vi "ProcessModbusUpdates.vi"(11 "MockInclinSettings":T1={"ModbusRxDataFIFO"="ModbusInclinRxDataFIFO", "ModbusTxDataFIFO"="ModbusInclinTxDataFIFO", "BufferUpdateFIFO"="MockInclinCommand", "InclinAngleMemory"="MockInlcinAngle"}) -> ()   [LabVIEW 2016]
uses:
  FPGAMockHPILC/DataTypes/MockHPModbusUpdateStates.ctl
  FPGAMockHPILC/FPGAMockHPILC.lvlib
  FPGAMockHPILC/DataTypes/MockHPModbusUpdateLoopData.ctl
  <vilib>/rvi/DataTransferAndStorage/Container/XNode/niFpgaContainer.xnode
  <vilib>/rvi/FIFO/Fifo_Resource/niFpgaFifoEmulationRefIn.vi
  <vilib>/rvi/FIFO/Fifo_Resource/nirvififoEmulationWrite.vi
  <vilib>/rvi/Memory/Memory_Emulation/nirvimemoryFastEmulation.vi
  <vilib>/rvi/Memory/Memory_Emulation/nirvimemoryEmulation.vi
  <vilib>/rvi/FIFO/Fifo_Resource/nirvififoEmulationRead.vi
  <vilib>/eio/EIOMethodNode/EIOMethodNode.xnode
  <vilib>/rvi/eio/common/nirviEmuTemplateMethod_errors.vi
  DataTypes/MockInclinSettings.ctl
  FPGAMockInclin.lvlib
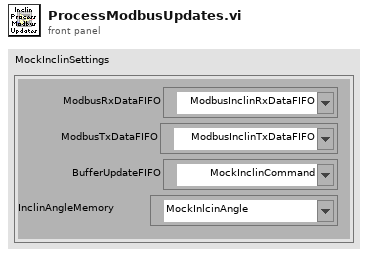
[diagram p1: front panel]
types:
  T1 = typedef "FPGAMockInclin.lvlib/MockInclinSettings.ctl" = cluster{"ModbusRxDataFIFO":refnum<k21>, "ModbusTxDataFIFO":refnum<k21>, "BufferUpdateFIFO":refnum<k21>, "InclinAngleMemory":refnum<k21>}
  T2 = typedef "FPGAMockHPILC.lvlib/MockHPModbusUpdateLoopData.ctl" = cluster{"ModbusUpdateLoopStates":T3, "Address":u8, "Function":u8, "ResponseLength":u8, "ResponseIndex":u8, "Index":u8, "Data":u16, "DelayTicks":u32}
  T3 = typedef "FPGAMockHPILC.lvlib/MockHPModbusUpdateStates.ctl" = enum16{"ReadModbusPort", "ProcessModbusData", "DelayMicroseconds", "WriteAddress", "WriteFunction", "WriteData", "WriteCRCLSB", "WriteCRCMSB", "WriteEndOfFrame", "CalculateCRC"}
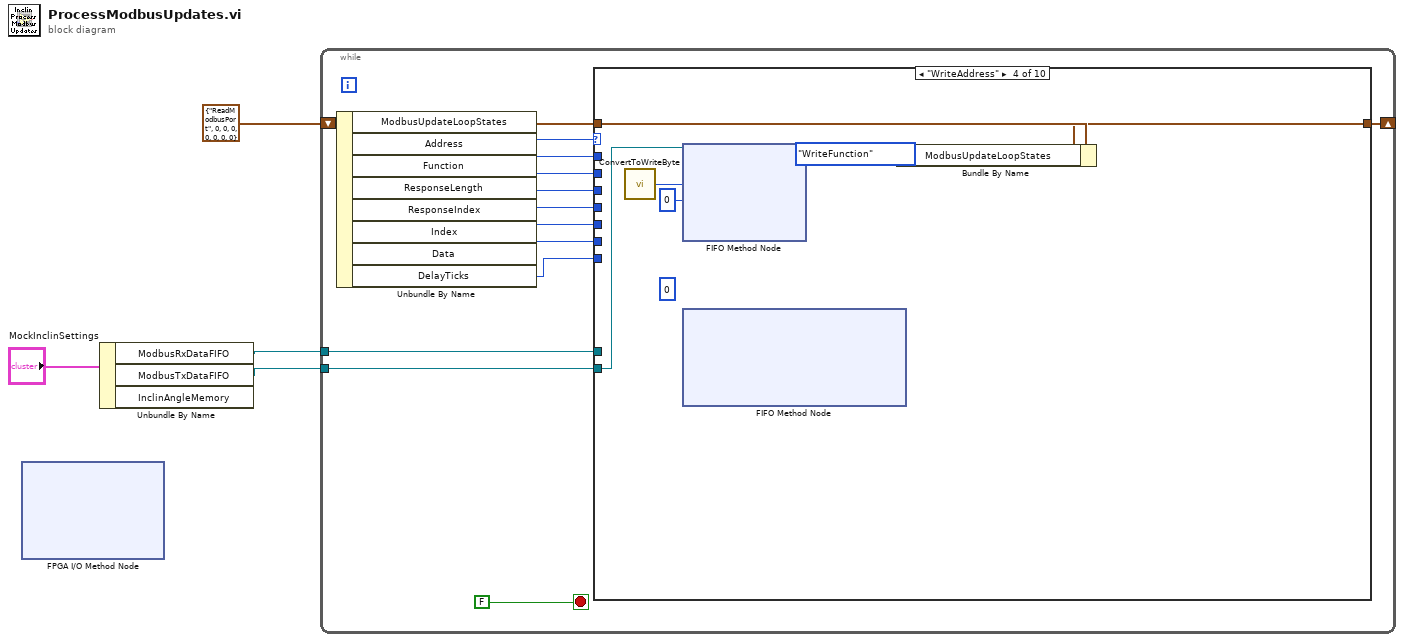
[diagram p0: block diagram]
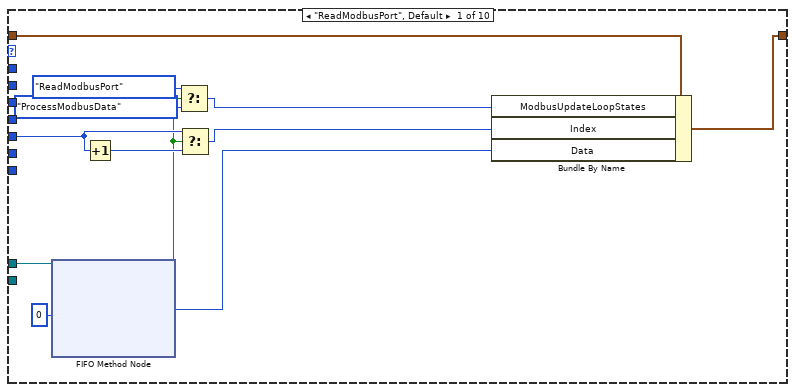
[diagram p2: hidden frame]
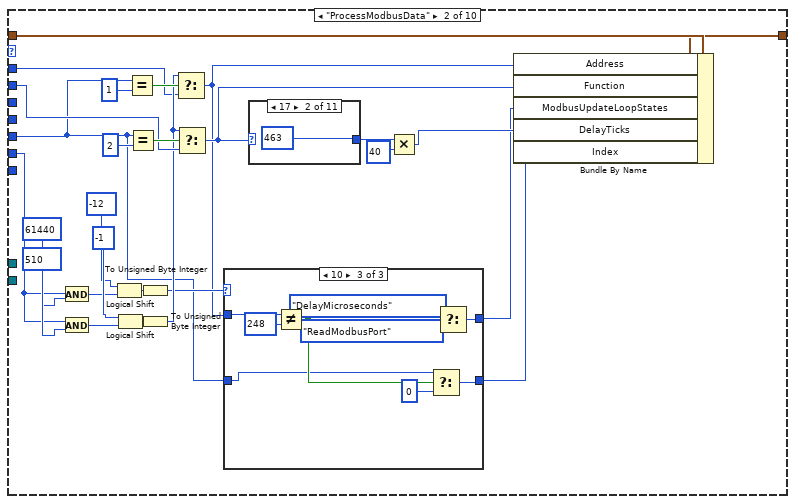
[diagram p3: hidden frame]
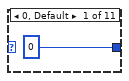
[diagram p4: hidden frame]
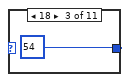
[diagram p5: hidden frame]
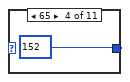
[diagram p6: hidden frame]
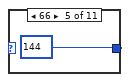
[diagram p7: hidden frame]
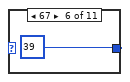
[diagram p8: hidden frame]
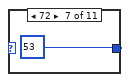
[diagram p9: hidden frame]
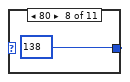
[diagram p10: hidden frame]
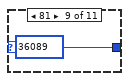
[diagram p11: hidden frame]
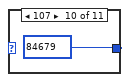
[diagram p12: hidden frame]
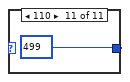
[diagram p13: hidden frame]
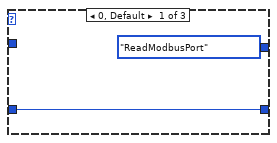
[diagram p14: hidden frame]
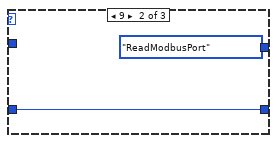
[diagram p15: hidden frame]
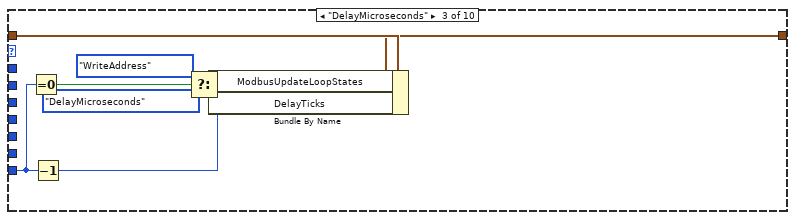
[diagram p16: hidden frame]
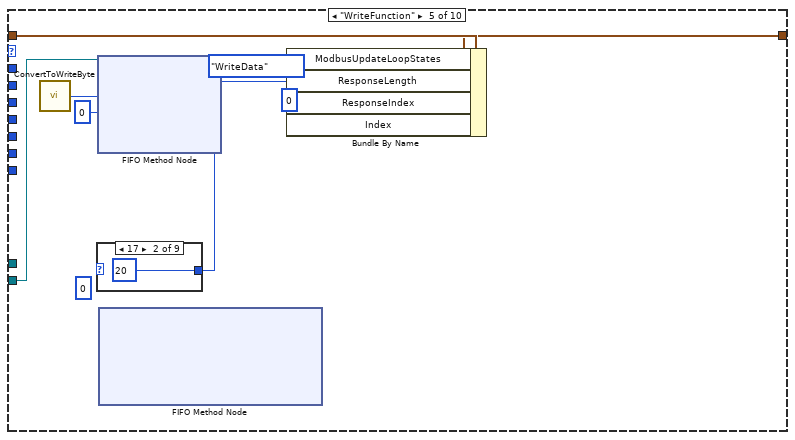
[diagram p17: hidden frame]
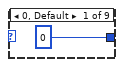
[diagram p18: hidden frame]
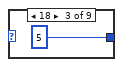
[diagram p19: hidden frame]
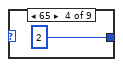
[diagram p20: hidden frame]
diagram:
  n1 = xnode "FPGA I/O Method Node"() -> ()  [unwired: 2 in, 3 out]
  n2 = Unbundle By Name("MockInclinSettings") -> ("ModbusRxDataFIFO"=w3:refnum<k21>, "ModbusTxDataFIFO"=w4:refnum<k21>)  [unwired: 1 out]
  n3 = while {
    shift-right: [w12] -> _
    shift-left: T2 {"ModbusUpdateLoopStates"=enum."ReadModbusPort", "Address"=0, "Function"=0, "ResponseLength"=0, "ResponseIndex"=0, "Index"=0, "Data"=0, "DelayTicks"=0} ("MockHPBufferUpdateLoopData") -> [w11]
    tunnel: w3 -> [w10]
    tunnel: w4 -> [w6]
    stop <- FALSE stop-if-true
    n4 = Unbundle By Name(w11) -> ("ModbusUpdateLoopStates"=w17:T3, "Address"=w16:u8, "Function"=w15:u8, "ResponseLength"=w14:u8, "ResponseIndex"=w13:u8, "Index"=w9:u8, "Data"=w8:u16, "DelayTicks"=w5:u32)
    n5 = case shown="\"WriteAddress\"" w17 {
      tunnel: w16 -> [_ w34 _ _ _ w128 _ _ _ _]
      tunnel: w15 -> [_ w43 _ _ _ w130 _ _ _ _]
      tunnel: w14 -> [_ _ _ _ _ w114 _ _ _ _]
      tunnel: w13 -> [_ _ _ _ _ w112 _ _ _ _]
      tunnel: [w20 w55 w87 w89 w97 w131 w171 w175 w184 w191] -> w12
      tunnel: w11 -> [w21 w56 w88 w91 w99 w132 w172 w176 w185 w196]
      tunnel: w10 -> [w29 _ _ _ _ _ _ _ _ _]
      tunnel: w9 -> [w24 w31 _ _ _ _ _ _ _ _]
      tunnel: w8 -> [_ w48 _ _ _ _ _ _ _ _]
      tunnel: w6 -> [_ _ _ w94 w102 w124 _ w174 w183 w195]
      tunnel: w5 -> [_ _ w82 _ _ _ _ _ _ _]
      frame "ReadModbusPort", Default {
        n6 = xnode ("FIFO Method Node")("Timeout"=0, "FIFO In"=w29) -> ("Element"=w18:u16, "Timed Out?"=w19:bool)  [unwired: 1 out]
        n7 = Increment(x=w24) -> (x+1=w25:u8)
        n8 = Select(t=MockHPModbusUpdateStates."ReadModbusPort", s=w19, f=MockHPModbusUpdateStates."ProcessModbusData") -> (s? t:f=w23:T3)
        n9 = Select(t=w24, s=w19, f=w25) -> (s? t:f=w22:u8)
        n10 = Bundle By Name(cluster=w21, "ModbusUpdateLoopStates"=w23, "Index"=w22, "Data"=w18) -> (w20:T2)
      }
      frame "ProcessModbusData" {
        n11 = And(x=w48, y=u16 61440) -> (x .and. y?=w50:u16)
        n12 = And(x=w48, y=u16 510) -> (x .and. y?=w53:u16)
        n13 = Logical Shift(y=i16 -12, x=w50) -> (x << y=w40:u16)
        n14 = Logical Shift(y=i16 -1, x=w53) -> (x << y=w42:u16)
        n15 = Equal?(x=w31, y=u8 1) -> (x = y?=w46:bool)
        n16 = Equal?(x=w31, y=u8 2) -> (x = y?=w45:bool)
        n17 = To Unsigned Byte Integer(number=w40) -> (unsigned 8bit integer=w39:u8)
        n18 = To Unsigned Byte Integer(number=w42) -> (unsigned 8bit integer=w41:u8)
        n19 = Select(t=w41, s=w46, f=w34) -> (s? t:f=w33:u8)
        n20 = Select(t=w41, s=w45, f=w43) -> (s? t:f=w38:u8)
        n21 = case shown="10" w39 {
          tunnel: [MockHPModbusUpdateStates."ReadModbusPort" ("f") MockHPModbusUpdateStates."ReadModbusPort" ("f") w80] -> w32
          tunnel: w33 -> [_ _ w76]
          tunnel: w31 -> [w68 w70 w74]
          tunnel: [w68 w70 w72] -> w30
          frame 0, Default {
          }
          frame 9 {
          }
          frame 10 {
            n22 = Not Equal?(x=w76, y=u8 248) -> (x != y?=w75:bool)
            n23 = Select(t=w74, s=w75, f=u8 0) -> (s? t:f=w72:u8)
            n24 = Select(t=MockHPModbusUpdateStates."DelayMicroseconds" ("f"), s=w75, f=MockHPModbusUpdateStates."ReadModbusPort") -> (s? t:f=w80:T3)
          }
        }
        n25 = case shown="17" w38 {
          tunnel: [u32 0 ("Count(uSec)") u32 463 ("Count(uSec)") u32 54 ("Count(uSec)") u32 152 ("Count(uSec)") u32 144 ("Count(uSec)") u32 39 ("Count(uSec)") u32 53 ("Count(uSec)") u32 138 ("Count(uSec)") u32 36089 ("Count(uSec)") u32 84679 ("Count(uSec)") u32 499 ("Count(uSec)")] -> w37
          frame 0, Default {
          }
          frame 17 {
          }
          frame 18 {
          }
          frame 65 {
          }
          frame 66 {
          }
          frame 67 {
          }
          frame 72 {
          }
          frame 80 {
          }
          frame 81 {
          }
          frame 107 {
          }
          frame 110 {
          }
        }
        n26 = Multiply(x=w37, y=u32 40) -> (x*y=w35:u32)
        n27 = Bundle By Name(cluster=w56, "Address"=w33, "Function"=w38, "ModbusUpdateLoopStates"=w32, "DelayTicks"=w35, "Index"=w30) -> (w55:T2)
      }
      frame "DelayMicroseconds" {
        n28 = Equal To 0?(x=w82) -> (x = 0?=w86:bool)
        n29 = Decrement(x=w82) -> (x-1=w81:u32)
        n30 = Select(t=MockHPModbusUpdateStates."WriteAddress", s=w86, f=MockHPModbusUpdateStates."DelayMicroseconds") -> (s? t:f=w85:T3)
        n31 = Bundle By Name(cluster=w88, "ModbusUpdateLoopStates"=w85, "DelayTicks"=w81) -> (w87:T2)
      }
      frame "WriteAddress" {
        (unwired) 0 ("Timeout")
        n32 = call "ConvertToWriteByte.vi"() -> ("Output"=w93:u16)  [unwired: 1 in]
        n33 = xnode ("FIFO Method Node")("Element"=w93, "Timeout"=0, "FIFO In"=w94) -> ()  [unwired: 2 out]
        n34 = xnode ("FIFO Method Node")() -> ()  [unwired: 3 in, 2 out]
        n35 = Bundle By Name(cluster=w91, "ModbusUpdateLoopStates"=MockHPModbusUpdateStates."WriteFunction") -> (w89:T2)
      }
      frame "WriteFunction" {
        (unwired) 0 ("Timeout")
        w95 = u8 0 ("ResponseIndex")
        n36 = call "ConvertToWriteByte.vi"() -> ("Output"=w101:u16)  [unwired: 1 in]
        n37 = case shown="17" {
          selector: _ -> [_ _ _ _ _ _ _ _ _]
          tunnel: [u8 0 ("ResponseLength") u8 20 ("ResponseLength") u8 5 ("ResponseLength") u8 2 ("ResponseLength") u8 9 ("ResponseLength") u8 9 ("ResponseLength") u8 1 ("ResponseLength") u8 1 ("ResponseLength") u8 96 ("ResponseLength")] -> w96
          frame 0, Default {
          }
          frame 17 {
          }
          frame 18 {
          }
          frame 65 {
          }
          frame 66 {
          }
          frame 67 {
          }
          frame 72 {
          }
          frame 80 {
          }
          frame 110 {
          }
        }
        n38 = xnode ("FIFO Method Node")("Element"=w101, "Timeout"=0, "FIFO In"=w102) -> ()  [unwired: 2 out]
        n39 = xnode ("FIFO Method Node")() -> ()  [unwired: 3 in, 2 out]
        n40 = Bundle By Name(cluster=w99, "ModbusUpdateLoopStates"=MockHPModbusUpdateStates."WriteData", "ResponseLength"=w96, "ResponseIndex"=w95, "Index"=w95) -> (w97:T2)
      }
      frame "WriteData" {
        n41 = Decrement(x=w128) -> (x-1=w129:u8)
        n42 = Multiply(x=w129, y=w114) -> (x*y=w127:u8)
        n43 = Add(x=w127, y=w112) -> (x+y=w126:u8)
        n44 = case shown="17" w130 {
          tunnel: w126 -> [_ w141 w145 w149 w153 w157 w161 w165 w169]
          tunnel: [u8 0 ("Data") w138 w142 w146 w150 w154 w158 w162 w166] -> w125
          tunnel: [FALSE TRUE TRUE TRUE TRUE TRUE TRUE TRUE TRUE] -> w117
          frame 0, Default {
          }
          frame 17 {
            n45 = xnode ("Memory Method Node")("Address"=w141) -> ("Data"=w139:u8)  [unwired: 1 in, 1 out]
            n46 = feedback-in #1(w139) -> ()
            n47 = feedback #1() -> (w138:u8)  [unwired: 1 in]
          }
          frame 18 {
            n48 = xnode ("Memory Method Node")("Address"=w145) -> ("Data"=w143:u8)  [unwired: 1 in, 1 out]
            n49 = feedback-in #2(w143) -> ()
            n50 = feedback #2() -> (w142:u8)  [unwired: 1 in]
          }
          frame 65 {
            n51 = xnode ("Memory Method Node")("Address"=w149) -> ("Data"=w147:u8)  [unwired: 1 in, 1 out]
            n52 = feedback-in #3(w147) -> ()
            n53 = feedback #3() -> (w146:u8)  [unwired: 1 in]
          }
          frame 66 {
            n54 = xnode ("Memory Method Node")("Address"=w153) -> ("Data"=w151:u8)  [unwired: 1 in, 1 out]
            n55 = feedback-in #4(w151) -> ()
            n56 = feedback #4() -> (w150:u8)  [unwired: 1 in]
          }
          frame 67 {
            n57 = xnode ("Memory Method Node")("Address"=w157) -> ("Data"=w155:u8)  [unwired: 1 in, 1 out]
            n58 = feedback-in #5(w155) -> ()
            n59 = feedback #5() -> (w154:u8)  [unwired: 1 in]
          }
          frame 72 {
            n60 = xnode ("Memory Method Node")("Address"=w161) -> ("Data"=w159:u8)  [unwired: 1 in, 1 out]
            n61 = feedback-in #6(w159) -> ()
            n62 = feedback #6() -> (w158:u8)  [unwired: 1 in]
          }
          frame 80 {
            n63 = xnode ("Memory Method Node")("Address"=w165) -> ("Data"=w163:u8)  [unwired: 1 in, 1 out]
            n64 = feedback-in #7(w163) -> ()
            n65 = feedback #7() -> (w162:u8)  [unwired: 1 in]
          }
          frame 110 {
            n66 = xnode ("Memory Method Node")("Address"=w169) -> ("Data"=w167:u8)  [unwired: 1 in, 1 out]
            n67 = feedback-in #8(w167) -> ()
            n68 = feedback #8() -> (w166:u8)  [unwired: 1 in]
          }
        }
        n69 = Increment(x=w112) -> (x+1=w119:u8)
        n70 = Increment(x=w114) -> (x+1=w113:u8)
        n71 = Equal To 0?(x=w112) -> (x = 0?=w118:bool)
        n72 = Equal?(x=w113, y=w119) -> (x = y?=w123:bool)
        n73 = Select(t=FALSE, s=w118, f=w117) -> (s? t:f=w116:bool)
        n74 = case shown="True" w116 {
          tunnel: w125 -> [_ _]
          tunnel: w124 -> [_ w133]
          frame False {
          }
          frame True {
            (unwired) 0 ("Timeout")
            n75 = call "ConvertToWriteByte.vi"() -> ("Output"=w134:u16)  [unwired: 1 in]
            n76 = xnode ("FIFO Method Node")("Element"=w134, "Timeout"=0, "FIFO In"=w133) -> ()  [unwired: 2 out]
            n77 = xnode ("FIFO Method Node")() -> ()  [unwired: 3 in, 2 out]
          }
        }
        n78 = Select(t=MockHPModbusUpdateStates."CalculateCRC", s=w123, f=MockHPModbusUpdateStates."WriteData") -> (s? t:f=w120:T3)
        n79 = Bundle By Name(cluster=w132, "ModbusUpdateLoopStates"=w120, "ResponseIndex"=w119) -> (w131:T2)
      }
      frame "CalculateCRC" {
        (unwired) 0 ("Timeout")
        (unwired) TRUE ("Element")
        n80 = xnode ("FIFO Write")() -> ()  [unwired: 1 in, 1 out]
        n81 = Bundle By Name(cluster=w172, "ModbusUpdateLoopStates"=MockHPModbusUpdateStates."WriteCRCLSB") -> (w171:T2)
      }
      frame "WriteCRCLSB" {
        (unwired) 0 ("Timeout")
        n82 = xnode ("FIFO Read")() -> ()  [unwired: 1 in, 1 out]
        n83 = case shown="False" {
          selector: _ -> [_ _]
          tunnel: w174 -> [w180 _]
          tunnel: [MockHPModbusUpdateStates."WriteCRCMSB" ("ModbusUpdateLoopStates") MockHPModbusUpdateStates."WriteCRCLSB" ("ModbusUpdateLoopStates")] -> w173
          frame False {
            n84 = call "ConvertToWriteByte.vi"() -> ("Output"=w179:u16)  [unwired: 1 in]
            n85 = xnode ("FIFO Write")("Element"=w179, "Timeout"=0, "FIFO In"=w180) -> ()  [unwired: 2 out]
          }
          frame True {
          }
        }
        n86 = Bundle By Name(cluster=w176, "ModbusUpdateLoopStates"=w173) -> (w175:T2)
      }
      frame "WriteCRCMSB" {
        (unwired) 0 ("Timeout")
        n87 = xnode ("FIFO Read")() -> ()  [unwired: 1 in, 1 out]
        n88 = case shown="False" {
          selector: _ -> [_ _]
          tunnel: w183 -> [w189 _]
          tunnel: [MockHPModbusUpdateStates."WriteEndOfFrame" ("ModbusUpdateLoopStates") MockHPModbusUpdateStates."WriteCRCMSB" ("ModbusUpdateLoopStates")] -> w182
          frame False {
            n89 = call "ConvertToWriteByte.vi"() -> ("Output"=w188:u16)  [unwired: 1 in]
            n90 = xnode ("FIFO Write")("Element"=w188, "Timeout"=0, "FIFO In"=w189) -> ()  [unwired: 2 out]
          }
          frame True {
          }
        }
        n91 = Bundle By Name(cluster=w185, "ModbusUpdateLoopStates"=w182) -> (w184:T2)
      }
      frame "WriteEndOfFrame" {
        n92 = xnode ("FIFO Write")("Element"=u16 8416, "Timeout"=0, "FIFO In"=w195) -> ()  [unwired: 2 out]
        n93 = Bundle By Name(cluster=w196, "ModbusUpdateLoopStates"=MockHPModbusUpdateStates."ReadModbusPort") -> (w191:T2)
      }
    }
  }
